vi "Elliptic Integral of the 1st kind.vi"   [LabVIEW 2017, in "NI_Gmath.lvlib"]
doc: "Computes the Legendre elliptic integral of the first kind. You must manually select the polymorphic instance you want to use."
uses:
  <vilib>/gmath/NI_Gmath.lvlib
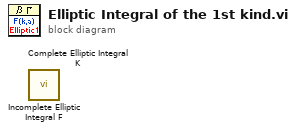
[diagram p0: block diagram]
diagram:
  n1 = call <vilib>:"Incomplete Elliptic Integral F.vi"() -> ()  [unwired: 11 in, 1 out]
  n2 = call <vilib>:"Complete Elliptic Integral K.vi"() -> ()  [unwired: 11 in, 1 out]
